vi "PH_StatusHandler.destructor.vi"(0 "i ref in":refnum<vi>, 5 "error in(no error)":errorcluster) -> (19 "error out":errorcluster)   [LabVIEW 2014, in "PH_StatusHandler.lvlib"]
doc: "This is the destructor of a class.\n\nLicense Agreement for this software:\n\nCopyright (C)\nGesellschaft für Schwerionenforschung, GSI\nPlanckstr. 1\n64291 Darmstadt\nGermany\n\nContact: D.Beck@gsi.de \n\nThis program is free software; you can redistribute it and/or modify it under the terms of the \nGNU General Public License as published by the Free Software Foundation; either version 2 of \nthe license, or (at your option) any later version.\n\nThis program is distributed in the hope that it will be useful, but WITHOUT ANY WARRANTY; \nwithout even the implied warranty of MERCHANTABILITY or FITNESS FOR A PARTICULAR PURPOSE. See the GNU General License for more details (http://www.gnu.org).\n\nGesellschaft für Schwerionenforschung, GSI\nPlanckstr. 1, 64291 Darmstadt, Germany\nFor all questions and ideas contact: M.Richter@gsi.de, H.Brand@gsi.de or D.Beck@gsi.de.\nLast update: 16-JUN-2004"
uses:
  PH_StatusHandler.lvlib
  PH_Class/PH_Class.lvlib
  lib.lib/DimLVEvent/LVDimInterface/LVDimInterface.lvlib
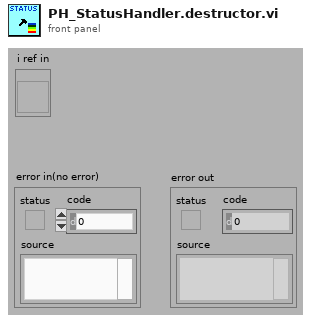
[diagram p1: front panel]
types:
  T1 = typedef "PH_StatusHandler.lvlib/PH_StatusHandler.i attribute.ctl" = cluster{"GUI Ref":refnum<vi>, "Value":T2, "Service ID":i32}
  T2 = typedef "PH_StatusHandler.lvlib/PH_StatusHandler.Status.ctl" = i16
  T3 = enum16{"SetAttribute", "GetAttribute", "CreateAttribute", "DestroyAttribute", "DestroyAllAtributes"}
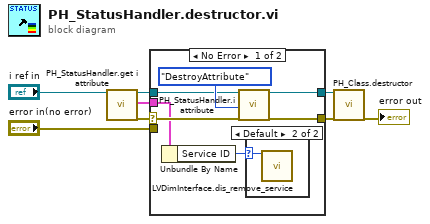
[diagram p0: block diagram]
diagram:
  n1 = call "PH_StatusHandler.get i attribute.vi"("i ref in"="i ref in") -> ("i ref out"=w6:refnum<vi>, "i attribute"=w1:T1, "error out"=w5:errorcluster)  [unwired: 16 in]
  n2 = case shown="No Error" w5 {
    selector: w5 -> [w11 _]
    tunnel: [w14 w17] -> w8
    tunnel: [w13 w18] -> w3
    tunnel: w6 -> [w12 w18]
    tunnel: "error in(no error)" -> [_ w17]
    tunnel: w1 -> [w10 _]
    frame No Error {
      n3 = Unbundle By Name(w10) -> ("Service ID"=w9:i32)
      n4 = call "PH_StatusHandler.i attribute.vi"("VI Refnum"=w12, "Action"=T3."DestroyAttribute", "error in (no error)"=w11) -> ("VI Refnum out"=w13:refnum<vi>, "error out"=w14:errorcluster)  [unwired: 14 in, 1 out]
      n5 = case shown="Default" w9 {
        selector: w9 -> [_ w16]
        frame -1 {
        }
        frame Default {
          n6 = call "LVDimInterface.dis_remove_service.vi"("my_serviceID"=w16) -> ()  [unwired: 18 in, 1 out]
        }
      }
    }
    frame Error {
    }
  }
  n7 = call "PH_Class.destructor.vi"("i ref in"=w3, "error in(no error)"=w8) -> ("error out"=→"error out":errorcluster)  [unwired: 17 in]
